vi "Build Menu Item for Pop-Up Menu.vi"(9 "Parent Menu":string, 10 "State":string, 11 "Menu Item Display Name":string) -> (3 "Cluster":T1)   [LabVIEW 2020]
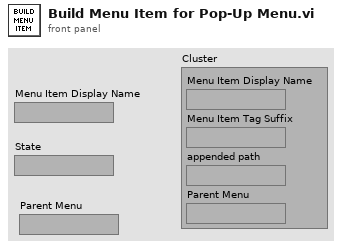
[diagram p1: front panel]
types:
  T1 = cluster{"Menu Item Display Name":string, "Menu Item Tag Suffix":string, "appended path":path, "Parent Menu":string}
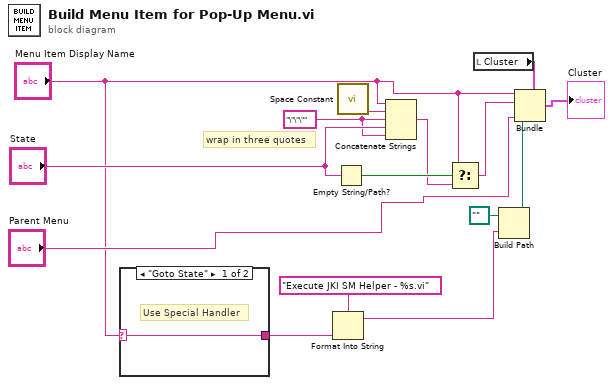
[diagram p0: block diagram]
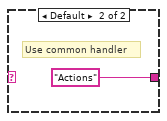
[diagram p2: hidden frame]
diagram:
  w1 = "\"\"\"" ("string")
  # "wrap in three quotes"
  n1 = case shown="\"Goto State\"" "Menu Item Display Name" {
    selector: "Menu Item Display Name" -> [w16 _]
    tunnel: [w16 "Actions" ("input 1")] -> w11
    frame "Goto State" {
      # "Use Special Handler"
    }
    frame Default {
      # "Use common handler"
    }
  }
  n2 = Format Into String(format string="Execute JKI SM Helper - %s.vi", w11) -> (resulting string=w10:string)  [unwired: 2 in, 1 out]
  n3 = Empty String/Path?(string/path="State") -> (empty?=w7:bool)
  n4 = call <vilib>:"Space Constant.vi"() -> ("String"=w2:string)
  n5 = Concatenate Strings("Menu Item Display Name", w2, w1, "State", w1) -> (w6:string)
  n6 = Select(t="Menu Item Display Name", s=w7, f=w6) -> (s? t:f=w5:string)
  n7 = local read "Cluster"() -> (w4:T1)
  n8 = Build Path(base path=path "..", name or relative path=w10) -> (appended path=w15:path)
  n9 = Bundle(cluster=w4, "Menu Item Display Name"="Menu Item Display Name", "Menu Item Tag Suffix"=w5, "appended path"=w15, "Parent Menu"="Parent Menu") -> (→"Cluster":T1)
